vi "Initialize (Remote).vi"(0 "device":refnum<k21>, 1 "Hostname/IP":string, 2 "Port":u16, 3 "https?":bool, 5 "Topology":string, 7 "topology suffix (none)":string, 9 "reset device (boolean value)":bool=TRUE, 11 "error in (no error)":errorcluster, 13 "username":string="admin", 14 "password":string) -> (4 "SLSC Switch out":refnum<class "SLSC Switch.lvclass">, 15 "error out":errorcluster)   [LabVIEW 2015, in "SLSC Switch.lvlib" / "SLSC Switch.lvclass"]
doc: "Returns a session handle used to identify the switch module in all subsequent driver calls and sets the topology of the switch module."
uses:
  SLSC Switch.lvclass
  <vilib>/National Instruments/SLSC Local or Remote Interface/SLSC Interface Class/SLSC Interface.lvclass
  <vilib>/National Instruments/SLSC Local or Remote Interface/SLSC Remote Interface Class/Initialize (Remote No Resource).vi
  <vilib>/National Instruments/SLSC Local or Remote Interface/SLSC Remote Interface Class/SLSC Remote.lvclass
  <vilib>/National Instruments/SLSC Local or Remote Interface/SLSC Remote Interface Class/Initialize (Remote NVMEM Area).vi
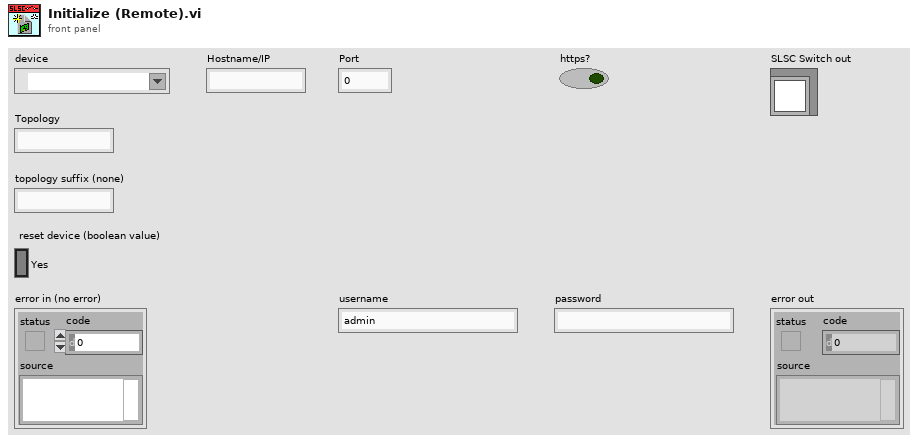
[diagram p1: front panel]
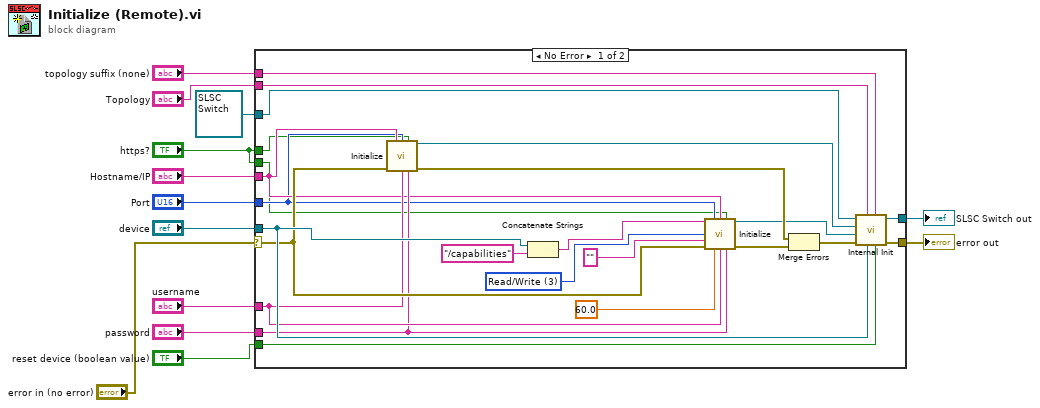
[diagram p0: block diagram]
diagram:
  n1 = case shown="No Error" "error in (no error)" {
    selector: "error in (no error)" -> [w30 w39]
    tunnel: [w36 w39] -> w11
    tunnel: refnum<class "SLSC Switch.lvclass"> refnum ("SLSC Switch in") -> [w37 w38]
    tunnel: "device" -> [w32 _]
    tunnel: "Topology" -> [w23 _]
    tunnel: "reset device (boolean value)" -> [w24 _]
    tunnel: [w35 w38] -> w12
    tunnel: "topology suffix (none)" -> [w34 _]
    tunnel: "username" -> [w19 _]
    tunnel: "password" -> [w18 _]
    tunnel: "Hostname/IP" -> [w17 _]
    tunnel: "Port" -> [w16 _]
    tunnel: "https?" -> [w15 _]
    tunnel: "https?" -> [w14 _]
    frame No Error {
      w22 = 3 items=["None"=0, "Read Only"=1, "Read/Write"=3] ("reservation access (Read/Write)")
      n2 = call-poly <vilib>:"Initialize.vi"("Hostname/IP"=w17, "Port"=w16, "https?"=w15, "error in (no error)"=w30, "username"=w19, "password"=w18) -> ("SLSC Remote out"=w25:refnum<class "SLSC Remote.lvclass">, "error out"=w29:errorcluster)  [unwired: 8 in]
      n3 = Concatenate Strings(w32, "/capabilities" ("string")) -> (w31:string)
      n4 = call-poly <vilib>:"Initialize.vi"("NVMEM areas"=w31, "Port"=w16, "Hostname/IP"=w17, "https?"=w14, "reservation access (Read/Write)"=w22, "reservation group"="", "error in (no error)"=w30, "connect timeout (60 sec)"=60.0, "username"=w19, "password"=w18) -> ("SLSC Remote out"=w26:refnum<class "SLSC Remote.lvclass">, "error out"=w28:errorcluster)  [unwired: 4 in]
      n5 = Merge Errors(w29, w28) -> (w27:errorcluster)
      n6 = call "Internal Init.vi"("reset device (boolean value)"=w24, "topology suffix (none)"=w34, "device"=w32, "Topology"=w23, "error in (no error)"=w27, "NVMEM Session"=w26, "No Resource Session"=w25, "SLSC Switch in"=w37) -> ("error out"=w36:errorcluster, "SLSC Switch out"=w35:refnum<class "SLSC Switch.lvclass">)  [unwired: 2 in]
    }
    frame Error {
    }
  }
  "error out" <- w11
  "SLSC Switch out" <- w12
